vi "Set Measurement Scale.vi"(6 "Log Scale (dB)":dbl=10.0 min=0.1 max=10.0 step=0.1 format="%.1f", 7 "Reference Level (dBm)":dbl=-10.0 min=-90.0 max=30.0 step=0.1 format="%.1f", 8 "error in (no error)":errorcluster, 9 "Span (nm)":dbl=1100.0 min=0.0 max=2250.0 step=0.5 format="%.3f", 10 "Center (nm)":dbl=1150.0 min=50.0 max=1700.0 step=0.5 format="%.3f", 11 "Optical Spectrum Analyzer in":refnum<class "Optical Spectrum Analyzer.lvclass">) -> (0 "error out":errorcluster, 3 "Optical Spectrum Analyzer out":refnum<class "Optical Spectrum Analyzer.lvclass">)   [LabVIEW 2018, in "Optical Spectrum Analyzer.lvlib" / "Optical Spectrum Analyzer.lvclass"]
uses:
  Optical Spectrum Analyzer.lvclass
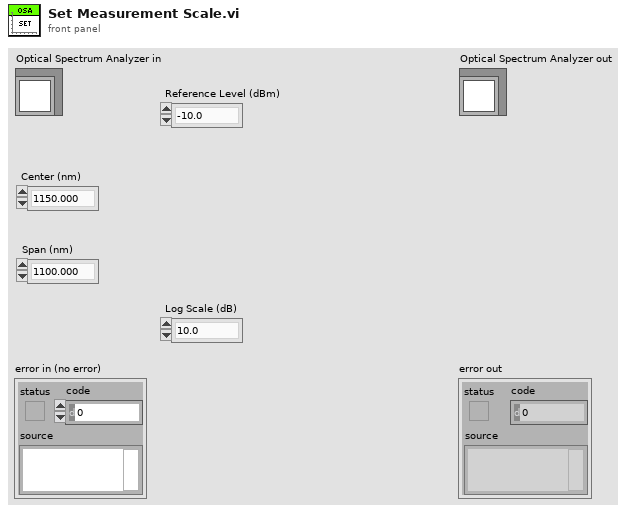
[diagram p1: front panel]
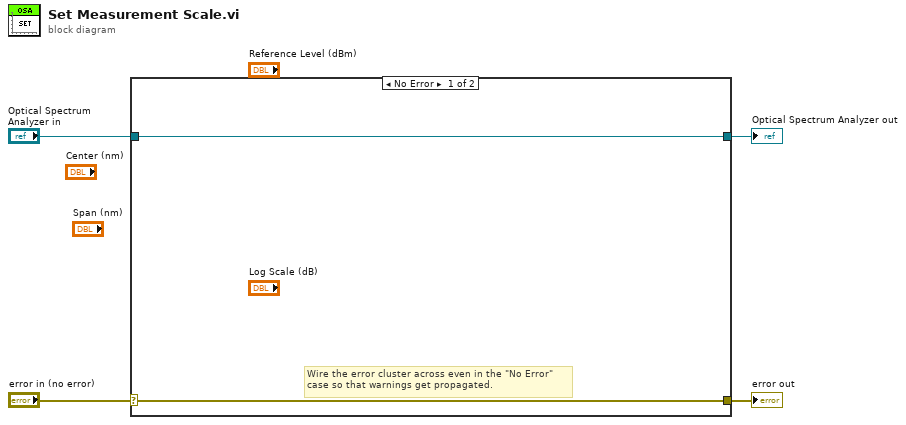
[diagram p0: block diagram]
diagram:
  n1 = case shown="No Error" "error in (no error)" {
    selector: "error in (no error)" -> [w5 w8]
    tunnel: [w5 w8] -> w3
    tunnel: [w6 w7] -> w1
    tunnel: "Optical Spectrum Analyzer in" -> [w6 w7]
    frame No Error {
      # "Wire the error cluster across even in the \"No Error\"\ncase so that warnings get propagated."
    }
    frame Error {
    }
  }
  "error out" <- w3
  "Optical Spectrum Analyzer out" <- w1
